vi "Drive Published Globals.vi"() -> ()   [LabVIEW 2015]
doc: "This is used primarily to publish values that other subsystems or user code may want to read periodically. It may also contain some settings such as debug switches or implementation selections that are independent of the operating mode of the subsystem."
uses:
  Support Code/labview-zmq/zmq_socket.lvclass
panel:
  in  "Distance to bin":dbl
  out "No Bin Detected":bool
  in  "Bin Angle":dbl
  in  "error in":errorcluster
  in  "socket in":refnum<class "zmq_socket.lvclass">
  in  "Encoder Right":dbl
  in  "Encoder Left":dbl
  # "Tip: The global is a good way publish state or\ninformational/debugging values.\nIt is not  advised that you put setpoint values here."
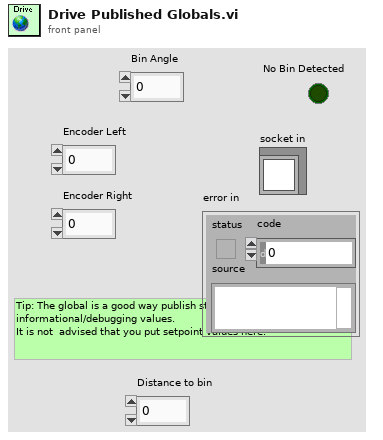
[diagram p1: front panel]
diagram:
